vi "testtest.vi"   [LabVIEW 2011]
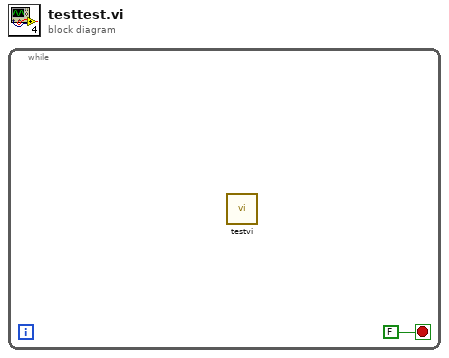
[diagram p0: block diagram]
diagram:
  n1 = while {
    stop <- FALSE stop-if-true
    n2 = call "testvi.vi"() -> ()  [unwired: 12 in]
  }
